vi "main.vi"() -> ()   [LabVIEW 2016]
uses:
  OptCtrl/OptCtrl.lvclass
  OptStateEsti/OptStateEsti.lvclass
panel:
  in  "Config File Name":string="optiPSSN_x00.ctrl"
  out "uk Array":dbl[](array[numeric])
  out "State in DOF 2":dbl[](array[numeric])
  in  "dofIdx":i32[](array[numeric])
  in  "State in DOF":dbl[](array[numeric])
  out "Qx Array":dbl[][](array[numeric])
  out "Matrix H":dbl[][](array[numeric])
  out "size(s)":i32[](array[numeric])
  out "F Matrix":dbl[][](array[numeric])
  in  "Filter Type":u16(ring) items=["ref", "u", "g", "r", "i", "z", "y"]
  in  "OptStateEsti in":refnum<class "OptStateEsti.lvclass">
  out "Range of DOF":dbl[](array[numeric])
  out "Authority":dbl[](array[numeric])
  in  "Gain":dbl=1.0
  in  "OptCtrl in":refnum<class "OptCtrl.lvclass">
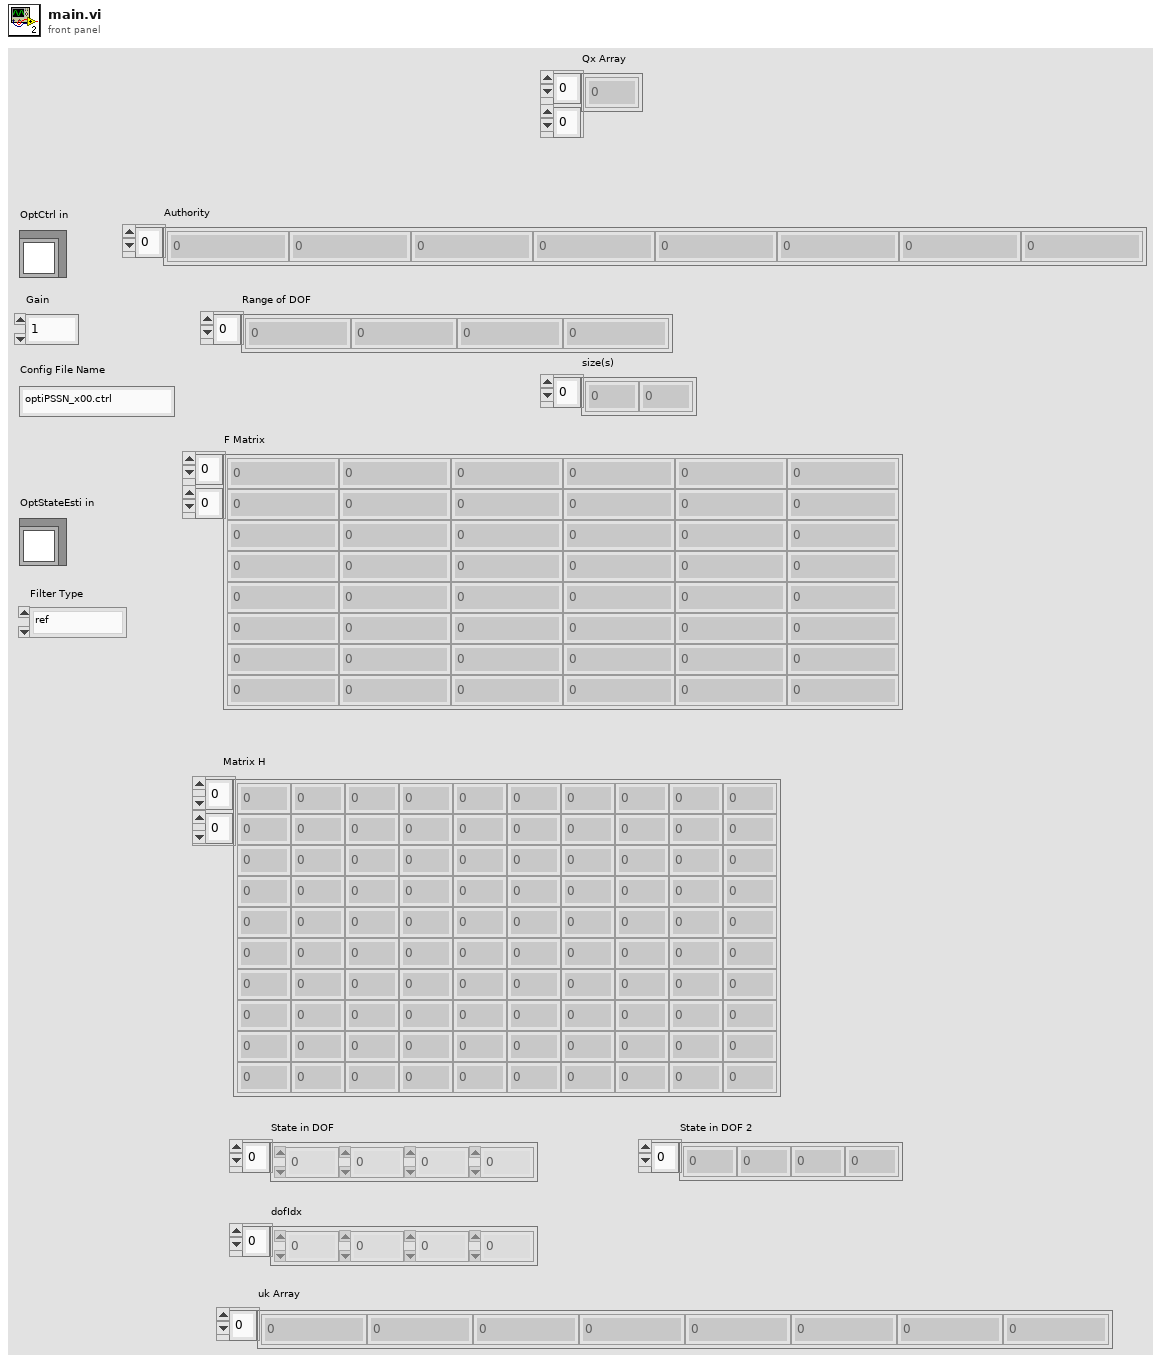
[diagram p1: front panel]
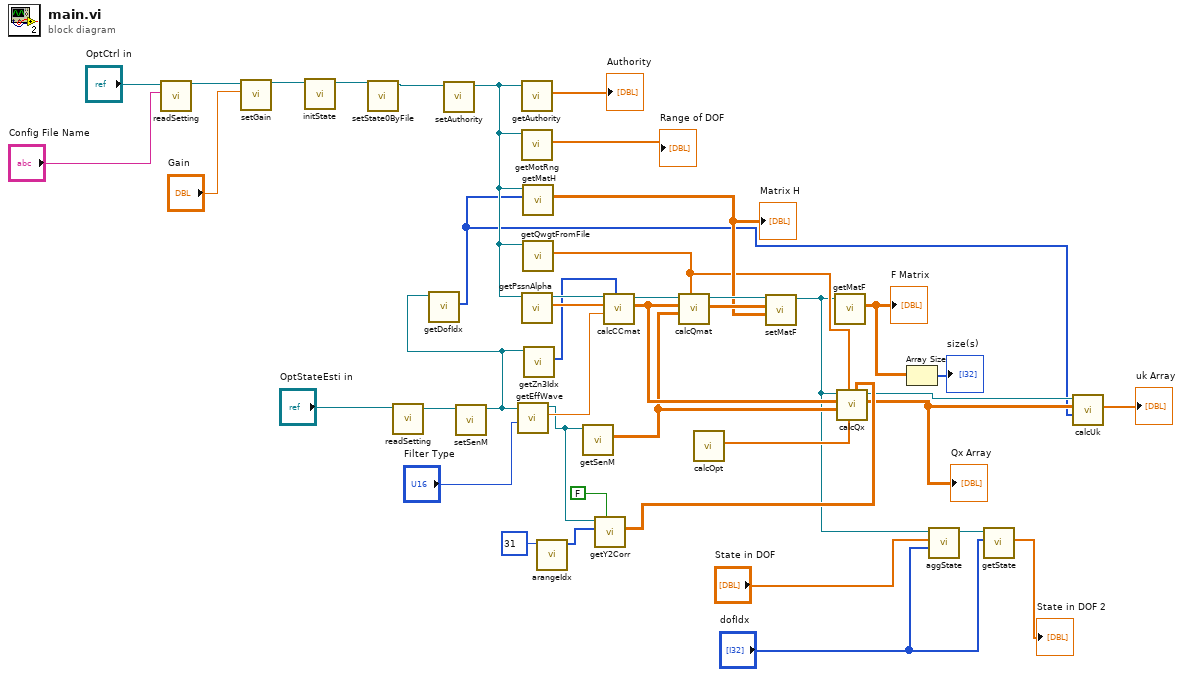
[diagram p0: block diagram]
diagram:
  n1 = call "readSetting.vi"("Config File Name"="Config File Name", "OptCtrl in"="OptCtrl in") -> ("OptCtrl out"=w9:refnum<class "OptCtrl.lvclass">)  [unwired: 8 in, 1 out]
  n2 = call "setGain.vi"("Gain"="Gain", "OptCtrl in"=w9) -> ("OptCtrl out"=w6:refnum<class "OptCtrl.lvclass">)  [unwired: 8 in, 1 out]
  n3 = call "initState.vi"("OptCtrl in"=w6) -> ("OptCtrl out"=w7:refnum<class "OptCtrl.lvclass">)  [unwired: 9 in, 1 out]
  n4 = call "setState0ByFile.vi"("OptCtrl in"=w7) -> ("OptCtrl out"=w14:refnum<class "OptCtrl.lvclass">)  [unwired: 9 in, 1 out]
  n5 = call "readSetting.vi"("OptStateEsti in"="OptStateEsti in") -> ("OptStateEsti out"=w37:refnum<class "OptStateEsti.lvclass">)  [unwired: 9 in, 1 out]
  n6 = call "setAuthority.vi"("OptCtrl in"=w14) -> ("OptCtrl out"=w28:refnum<class "OptCtrl.lvclass">)  [unwired: 9 in, 1 out]
  n7 = call "setSenM.vi"("OptStateEsti in"=w37) -> ("OptStateEsti out"=w27:refnum<class "OptStateEsti.lvclass">)  [unwired: 9 in, 1 out]
  n8 = call "getDofIdx.vi"("OptStateEsti in"=w27) -> ("dofIdx"=w3:i32[])  [unwired: 8 in, 2 out]
  n9 = call "getEffWave.vi"("Filter Type"="Filter Type", "OptStateEsti in"=w27) -> ("Effective Wavelength  (um)"=w35:dbl, "OptStateEsti out"=w23:refnum<class "OptStateEsti.lvclass">)  [unwired: 7 in, 1 out]
  n10 = call "getAuthority.vi"("OptCtrl in"=w28) -> ("Authority"=→"Authority":dbl[])  [unwired: 8 in, 2 out]
  n11 = call "getMotRng.vi"("OptCtrl in"=w28) -> ("Range of DOF"=→"Range of DOF":dbl[])  [unwired: 8 in, 2 out]
  n12 = call "getPssnAlpha.vi"("OptCtrl in"=w28) -> ("PSSN Alpha"=w33:dbl[], "OptCtrl out"=w34:refnum<class "OptCtrl.lvclass">)  [unwired: 8 in, 1 out]
  n13 = call "getMatH.vi"("dofIdx"=w3, "OptCtrl in"=w28) -> ("Matrix H"=w26:dbl[][])  [unwired: 7 in, 2 out]
  "Matrix H" <- w26
  n14 = call "getQwgtFromFile.vi"("OptCtrl in"=w28) -> ("Wgt of Q"=w17:dbl[])  [unwired: 8 in, 2 out]
  n15 = call "getZn3Idx.vi"("OptStateEsti in"=w27) -> ("zn3Idx"=w29:i32[])  [unwired: 8 in, 2 out]
  n16 = call "arangeIdx.vi"("Number"=31) -> ("Idx Array"=w21:i32[])  [unwired: 10 in]
  n17 = call "getSenM.vi"("OptStateEsti in"=w23) -> ("Sen M"=w18:dbl[][][])  [unwired: 8 in, 2 out]
  n18 = call "getY2Corr.vi"("In nx1 Row"=FALSE, "Field Idx"=w21, "OptStateEsti in"=w23) -> ("y2c Array"=w16:dbl[][])  [unwired: 6 in, 2 out]
  n19 = call "calcCCmat.vi"("zn3Idx"=w29, "Effective Wavelength"=w35, "PSSN Alpha"=w33, "OptCtrl in"=w34) -> ("CC Matrix"=w19:dbl[][], "OptCtrl out"=w32:refnum<class "OptCtrl.lvclass">)  [unwired: 5 in, 1 out]
  n20 = call "calcQmat.vi"("Weighting of Field Point"=w17, "Sen M"=w18, "CC Matrix"=w19, "OptCtrl in"=w32) -> ("Q Matrix"=w30:dbl[][], "OptCtrl out"=w31:refnum<class "OptCtrl.lvclass">)  [unwired: 5 in, 1 out]
  n21 = call "calcOpt.vi"() -> ("Optical State"=w15:dbl[])  [unwired: 11 in]
  n22 = call "setMatF.vi"("Matrix H"=w26, "Q Matrix"=w30, "OptCtrl in"=w31) -> ("OptCtrl out"=w8:refnum<class "OptCtrl.lvclass">)  [unwired: 7 in, 1 out]
  n23 = call "getMatF.vi"("OptCtrl in"=w8) -> ("F Matrix"=w25:dbl[][])  [unwired: 8 in, 2 out]
  "F Matrix" <- w25
  n24 = call "calcQx.vi"("y2 Matrix"=w16, "Optical State"=w15, "Weighting of Field Point"=w17, "Sen M"=w18, "CC Matrix"=w19, "OptCtrl in"=w8) -> ("Qx Array"=w4:dbl[][], "OptCtrl out"=w5:refnum<class "OptCtrl.lvclass">)  [unwired: 3 in, 1 out]
  "Qx Array" <- w4
  n25 = Array Size(array=w25) -> (size(s)=→"size(s)":i32[])
  n26 = call "aggState.vi"("dofIdx"="dofIdx", "State in DOF"="State in DOF", "OptCtrl in"=w8) -> ("OptCtrl out"=w12:refnum<class "OptCtrl.lvclass">)  [unwired: 7 in, 1 out]
  n27 = call "getState.vi"("dofIdx"="dofIdx", "OptCtrl in"=w12) -> ("State in DOF"=→"State in DOF 2":dbl[])  [unwired: 7 in, 2 out]
  n28 = call "calcUk.vi"("dofIdx"=w3, "Qx Array"=w4, "OptCtrl in"=w5) -> ("uk Array"=→"uk Array":dbl[])  [unwired: 6 in, 2 out]
